vi "TCP - Clear All Buffered Data.vi"(8 "error in":errorcluster, 11 "TCP Network Connection in":refnum<k5>) -> (0 "error out":errorcluster, 3 "TCP Network Connection out":refnum<k5>)   [LabVIEW 2020]
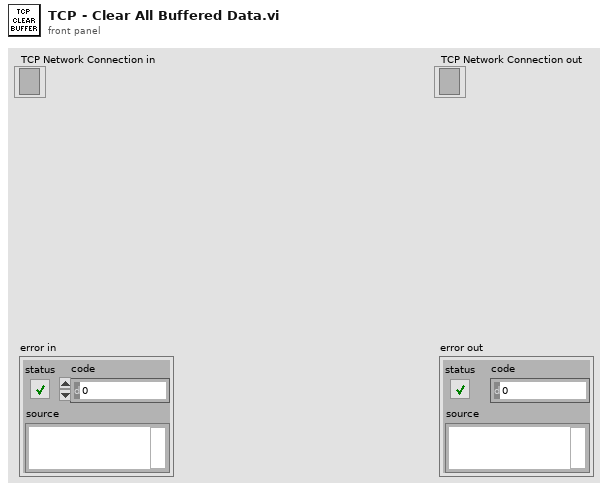
[diagram p1: front panel]
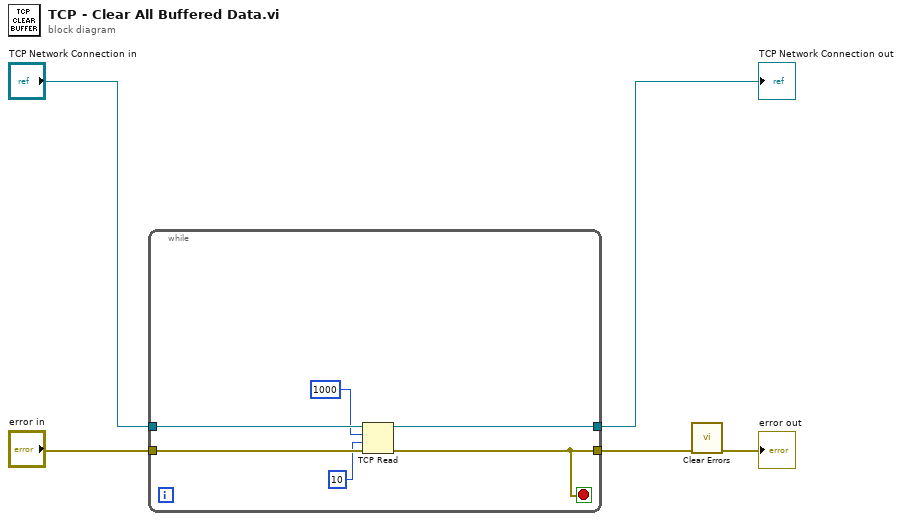
[diagram p0: block diagram]
diagram:
  n1 = while {
    tunnel: "error in" -> [w11]
    tunnel: [w6] -> w2
    tunnel: "TCP Network Connection in" -> [w10]
    tunnel: [w9] -> w3
    stop <- w6 stop-if-true
    n2 = TCP Read(connection ID=w10, bytes to read=1000, error in (no error)=w11, 9:10 ("timeout ms (25000)")) -> (connection ID out=w9:refnum<k5>, error out=w6:errorcluster)  [unwired: 1 in, 1 out]
  }
  "TCP Network Connection out" <- w3
  n3 = call <vilib>:"Clear Errors.vi"("error in (no error)"=w2) -> ("error out"=→"error out":errorcluster)  [unwired: 5 in, 1 out]
